vi "Streamline2017.vi"   [LabVIEW 2013]
uses:
  ModeType.ctl
  <vilib>/Heliosphere Research LLC/Advanced Plotting Toolkit/Advanced Plotting Toolkit.lvlib
types:
  T1 = typedef "ModeType.ctl" = enum16{"Normal", "Expected Failure", "Skipped", "Broken"}
  T2 = typedef "Advanced Plotting Toolkit.lvlib/PlotID.ctl" = i32
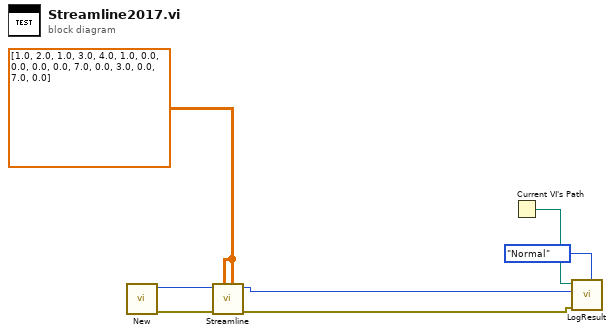
[diagram p0: block diagram]
diagram:
  w4 = dbl[][] [[1.0, 2.0, 1.0, 3.0], [4.0, 1.0, 0.0, 0.0], [0.0, 0.0, 7.0, 0.0], [3.0, 0.0, 7.0, 0.0]] ("Data")
  n1 = call <vilib>:"New.vi"() -> ("error out"=w5:errorcluster, "Plot ID"=w6:T2)  [unwired: 10 in]
  n2 = call <vilib>:"Streamline.vi"("Y Vector Component"=w4, "X Vector Component"=w4, "error in (no error)"=w5, "Plot ID"=w6) -> ("error out"=w1:errorcluster, "Plot ID Out"=w2:T2)  [unwired: 6 in]
  n3 = Current VI's Path() -> (path=w7:path)
  n4 = call "LogResult.vi"("Mode"=ModeType."Normal", "Test Result"=w1, "Test Artifact"=w2, "VI Path"=w7) -> ()  [unwired: 8 in]
